vi "SignalGen (SubVI).vi"(0 "phasex":dbl, 4 "2X%1X":dbl, 5 "Y":dbl=1.0 format="%0.2p", 6 "X":dbl=1.0 format="%0.2p", 7 "freq1X":dbl=20.0 format="%0.2p") -> (1 "Waveform 3":waveform(dbl)(graph)={"t0"=timestamp(15 s since 1904-01-01), "dt"=0.001, "Y"=[]}, 2 "Waveform 2":waveform(dbl)(graph), 3 "Waveform":waveform(dbl)(graph)={"t0"=timestamp(15 s since 1904-01-01), "dt"=0.001, "Y"=[]})   [LabVIEW 2012]
uses:
  <vilib>/measure/NI_MABase.lvlib
panel:
  in  "offset 3":dbl format="%0.2p"
  in  "reset signal 3":bool
  in  "signal type 3":T1(ring)
  in  "phase 3":dbl=10.0 format="%0.2f"
  in  "sampling info 3":cluster{"Fs":dbl, "#s":dbl}={"Fs"=10240.0, "#s"=1000.0} {"Fs" format="%0.2p"}
  in  "duty cycle (%) 3":dbl=50.0 format="%0.2f"
  in  "offset 2":dbl format="%0.2p"
  in  "reset signal 2":bool
  in  "signal type 2":T1(ring)
  in  "phase 2":dbl=100.0 format="%0.2f"
  in  "sampling info 2":cluster{"Fs":dbl, "#s":dbl}={"Fs"=10240.0, "#s"=1000.0} {"Fs" format="%0.2p"}
  in  "duty cycle (%) 2":dbl=50.0 format="%0.2f"
  in  "offset":dbl format="%0.2p"
  in  "reset signal":bool
  in  "signal type":T1(ring)=enum."Square Wave"
  in  "amplitude":dbl=1.0 format="%0.2p"
  in  "phase":dbl format="%0.2f"
  in  "sampling info":cluster{"Fs":dbl, "#s":dbl}={"Fs"=10240.0, "#s"=1000.0} {"Fs" format="%0.2p"}
  in  "duty cycle (%)":dbl=3.0 format="%0.2f"
  # "RANK"
  # "RANK"
  # "RANK"
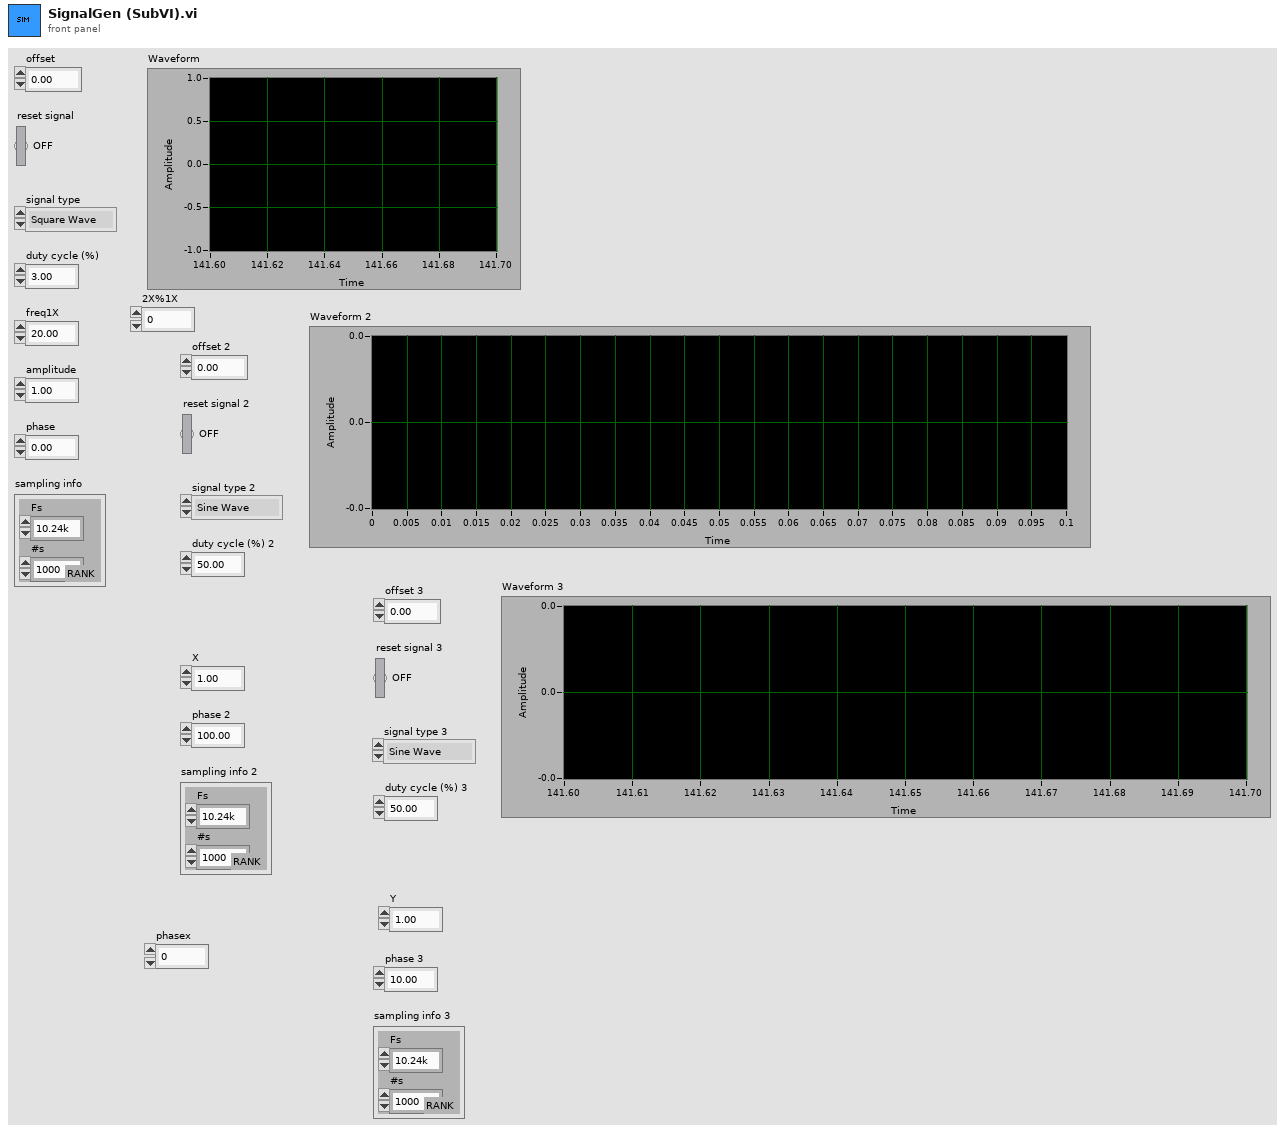
[diagram p1: front panel]
types:
  T1 = enum16{"Sine Wave", "Triangle Wave", "Square Wave", "Sawtooth Wave"}
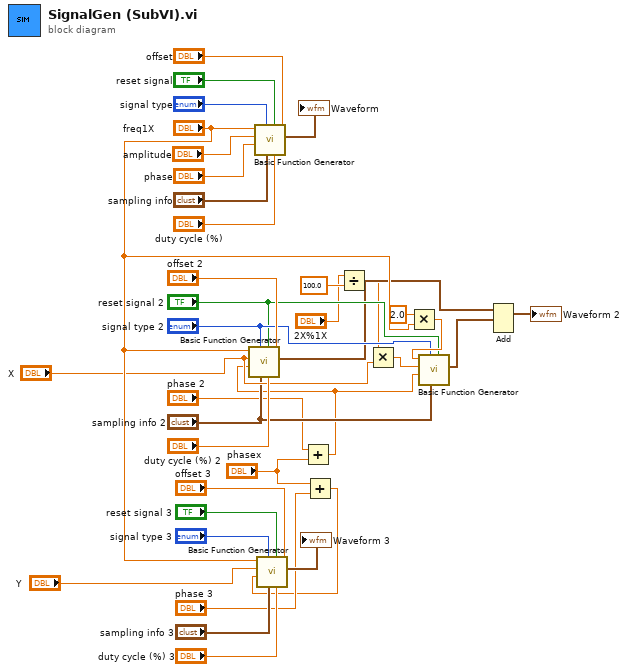
[diagram p0: block diagram]
diagram:
  n1 = call <vilib>:"Basic Function Generator.vi"("offset"="offset", "square wave duty cycle (%)"="duty cycle (%)", "reset signal"="reset signal", "sampling info"="sampling info", "signal type"="signal type", "phase"="phase", "amplitude"="amplitude", "frequency"="freq1X") -> ("signal out"=→"Waveform":waveform(dbl))  [unwired: 1 in, 2 out]
  n2 = Add(x="phase 2", y="phasex") -> (x+y=w4:dbl)
  n3 = call <vilib>:"Basic Function Generator.vi"("offset"="offset 2", "square wave duty cycle (%)"="duty cycle (%) 2", "reset signal"="reset signal 2", "sampling info"="sampling info 2", "signal type"="signal type 2", "phase"=w4, "amplitude"="X", "frequency"="freq1X") -> ("signal out"=w11:waveform(dbl))  [unwired: 1 in, 2 out]
  n4 = Add(x="phasex", y="phase 3") -> (x+y=w1:dbl)
  n5 = call <vilib>:"Basic Function Generator.vi"("offset"="offset 3", "square wave duty cycle (%)"="duty cycle (%) 3", "reset signal"="reset signal 3", "sampling info"="sampling info 3", "signal type"="signal type 3", "phase"=w1, "amplitude"="Y", "frequency"="freq1X") -> ("signal out"=→"Waveform 3":waveform(dbl))  [unwired: 1 in, 2 out]
  n6 = Divide(x="2X%1X", y=100.0) -> (x/y=w6:dbl)
  n7 = Multiply(x=w6, y="X") -> (x*y=w16:dbl)
  n8 = Multiply(x=2.0, y="freq1X") -> (x*y=w19:dbl)
  n9 = call <vilib>:"Basic Function Generator.vi"("reset signal"="reset signal 2", "sampling info"="sampling info 2", "signal type"="signal type 2", "phase"=w4, "amplitude"=w16, "frequency"=w19) -> ("signal out"=w10:waveform(dbl))  [unwired: 3 in, 2 out]
  n10 = Add(1:w10, 2:w11) -> (0:→"Waveform 2":waveform(dbl))  [unwired: 1 in, 1 out]
